vi "Geometry_Util_Delta.vi"() -> (3 "Delta":dbl)   [LabVIEW 2019]
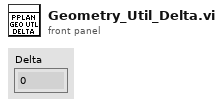
[diagram p1: front panel]
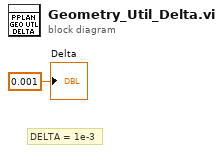
[diagram p0: block diagram]
diagram:
  # "DELTA = 1e-3"
  "Delta" <- 0.001 ("Delta")
